vi "get number of physical channels.vi"(8 "error in (no error)":errorcluster, 11 "device type":T1=enum."LAN") -> (0 "error out":errorcluster, 3 "number of physical channels":u8)   [LabVIEW 2024, in "atsj peakcan basic.lvlib"]
doc: "Gets the maximum <b>number of physical channels</b> supported by the specified <b>device type</b> / bus type."
uses:
  atsj peakcan basic.lvlib
  device type.ctl
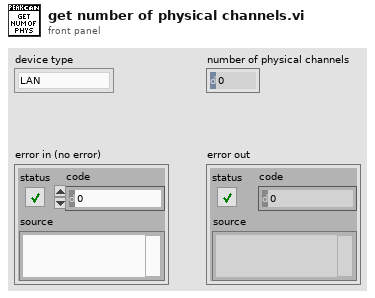
[diagram p1: front panel]
types:
  T1 = typedef "atsj peakcan basic.lvlib/device type.ctl" = enum8{"ISA", "DNG", "PCI", "USB", "PCC", "LAN"}
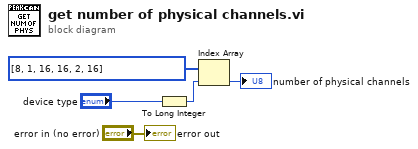
[diagram p0: block diagram]
diagram:
  n1 = To Long Integer(number="device type") -> (32bit integer=w4:i32)
  n2 = Index Array(array=u8[] [8, 1, 16, 16, 2, 16] ("Array"), index=w4) -> (element=→"number of physical channels":u8)
  "error out" <- "error in (no error)"
